vi "test1_new.vi"() -> ()   [LabVIEW 2014]
uses:
  <vilib>/vision/Image Controls.llb/IMAQ Image.ctl
  <resource>/objmgr/IMAQImage.rc
  EmergentCameraC/EmergentCameraC.lvlib
panel:
  in  "New Image":T1
  in  "stop":bool
  out "Image":T1(plugin-control)
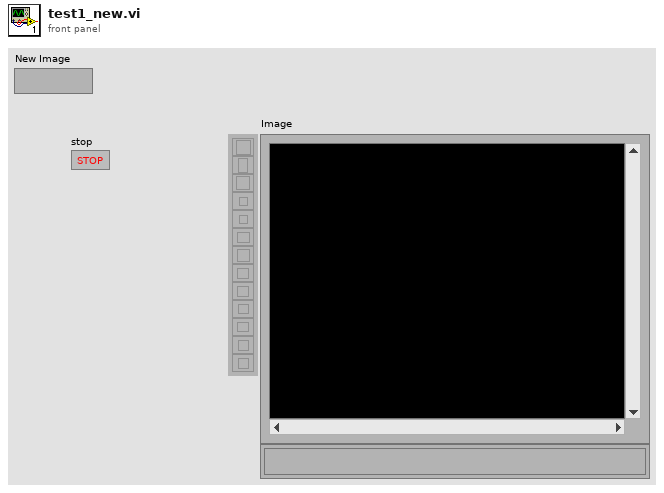
[diagram p1: front panel]
types:
  T1 = typedef "IMAQ Image.ctl" = refnum<image>
  T2 = typedef "Image Type" = u32
  T3 = enum32{"Map Pixel Pointer", "Unmap Pixel Pointer", "Get Pixels Infos"}
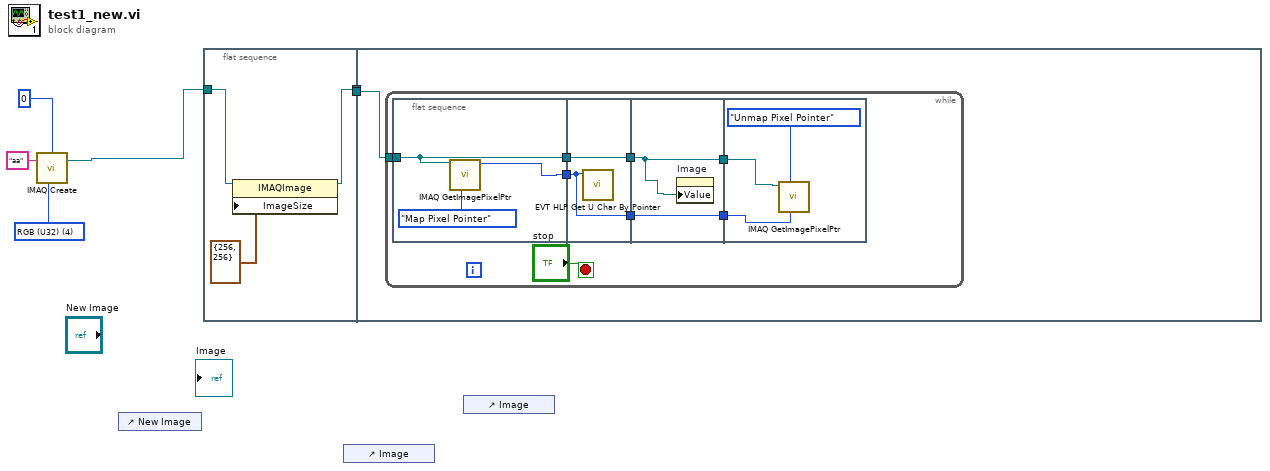
[diagram p0: block diagram]
diagram:
  w3 = T2 4 items=["Grayscale (U8)", "Grayscale (I16)", "Grayscale (SGL)", "Complex (CSG)", "RGB (U32)", "HSL (U32)", "RGB (U64)", "Grayscale (U16)"] ("Image Type")
  n1 = call "IMAQ Create"("Border Size"=0, "Image Name"="aa", "Image Type"=w3) -> ("New Image"=w5:T1)  [unwired: 2 in, 1 out]
  n2 = control-ref of="New Image"() -> ()  [unwired: 1 out]
  n3 = flat-sequence {
    tunnel: w5 -> [w8]
    tunnel: [w7] -> w1
    tunnel: w1 -> [w9]
    frame #0 {
      n4 = property class="IMAQImage"(reference=w8, "ImageSize"=cluster{"x":i32, "y":i32} {"x"=256, "y"=256} ("Image Size")) -> (reference out=w7:T1)  [unwired: 1 in, 1 out]
    }
    frame #1 {
      n5 = while {
        tunnel: w9 -> [w15]
        stop <- "stop" stop-if-true
        n6 = flat-sequence {
          tunnel: w15 -> [w19]
          tunnel: [w18] -> w14
          tunnel: [w19] -> w13
          tunnel: [w22] -> w16
          tunnel: w14 -> [w21]
          tunnel: w13 -> [w22]
          tunnel: [w21] -> w11
          tunnel: w16 -> [w23]
          tunnel: [w24] -> w12
          tunnel: w11 -> [w24]
          tunnel: [w23] -> w10
          tunnel: w12 -> [w26]
          tunnel: w10 -> [w25]
          frame #0 {
            n7 = call "IMAQ GetImagePixelPtr"("Function"=T3."Map Pixel Pointer", "Image"=w19) -> ("Pixel Pointer out"=w18:u64)  [unwired: 4 in, 5 out]
          }
          frame #1 {
            n8 = call "EVT HLP Get U Char By Pointer.vi"("ptr"=w21) -> ()  [unwired: 10 in, 1 out]
          }
          frame #2 {
            n9 = property on="Image" class="ImageControl"("Value"=w23) -> ()  [unwired: 2 in, 2 out]
          }
          frame #3 {
            n10 = call "IMAQ GetImagePixelPtr"("Pixel Pointer in"=w26, "Function"=T3."Unmap Pixel Pointer", "Image"=w25) -> ()  [unwired: 3 in, 6 out]
          }
        }
      }
    }
  }
  n11 = control-ref of="Image"() -> ()  [unwired: 1 out]
  n12 = control-ref of="Image"() -> ()  [unwired: 1 out]
